vi "VerifyPartialClusterStrings.vi"(10 "Input String":string, 11 "Cluster":T1) -> (3 "Values The Expected Values":bool)   [LabVIEW 2010]
panel:
  in  "String 2":string="This is a default value"
  in  "Array 2":string[](array[string])=["Has ", "More ", "Default ", "Values"]
  in  "Array 1":string[](array[string])=["Has ", "Default ", "Values"]
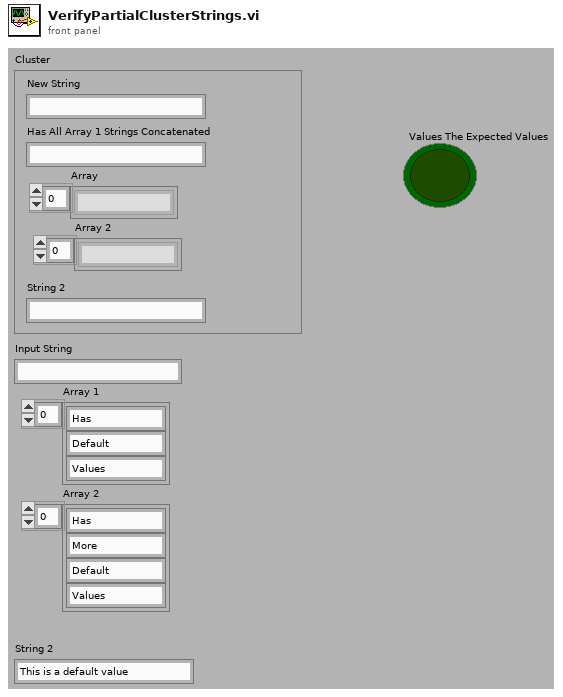
[diagram p1: front panel]
types:
  T1 = cluster{"New String":string, "Has All Array 1 Strings Concatenated":string, "Array":string[], "Array 2":string[], "String 2":string}
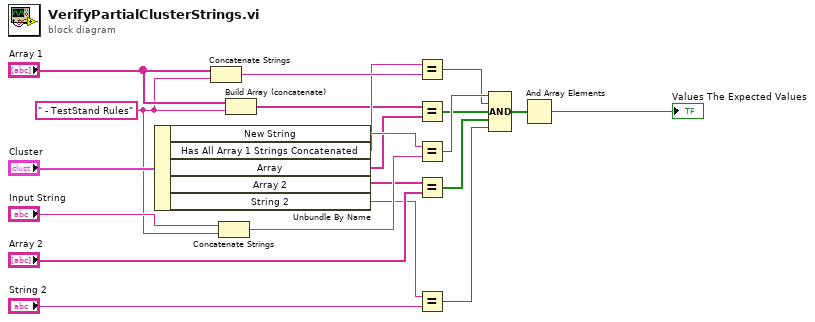
[diagram p0: block diagram]
diagram:
  w14 = " - TestStand Rules"
  n1 = Unbundle By Name("Cluster") -> ("New String"=w19:string, "Has All Array 1 Strings Concatenated"=w16:string, "Array"=w12:string[], "Array 2"=w11:string[], "String 2"=w9:string)
  n2 = Concatenate Strings("Array 1", w14) -> (w17:string)
  n3 = Concatenate Strings("Input String", w14) -> (w18:string)
  n4 = Build Array (concatenate)("Array 1", w14) -> (w13:string[])
  n5 = Equal?(x=w16, y=w17) -> (x = y?=w6:bool)
  n6 = Equal?(x=w13, y=w12) -> (x = y?=w5:bool[])
  n7 = Equal?(x=w19, y=w18) -> (x = y?=w7:bool)
  n8 = Equal?(x=w11, y="Array 2") -> (x = y?=w4:bool[])
  n9 = Equal?(x=w9, y="String 2") -> (x = y?=w3:bool)
  n10 = Compound Arithmetic op=AND(w7, w6, w5, w4, w3) -> (w2:bool[])
  n11 = And Array Elements(Boolean array=w2) -> (logical AND=→"Values The Expected Values":bool)
